vi "GetPulsePositionsByName.vi"(8 "error in (no error)":errorcluster, 10 "Channel Name":string, 11 "Pulse Positions Array":T1[](array[typedef])) -> (0 "error out":errorcluster, 1 "Pulse Positions":T1, 2 "Found?":bool, 3 "Pulse Positions Array Out":T1[](array[typedef]))   [LabVIEW 2017]
uses:
  <vilib>/addons/InsightCM/Utilities/Analysis/Shared/controls/PulsePositions.ctl
  <vilib>/addons/InsightCM/Utilities/Analysis/Shared/AnalysisHelper.lvlib
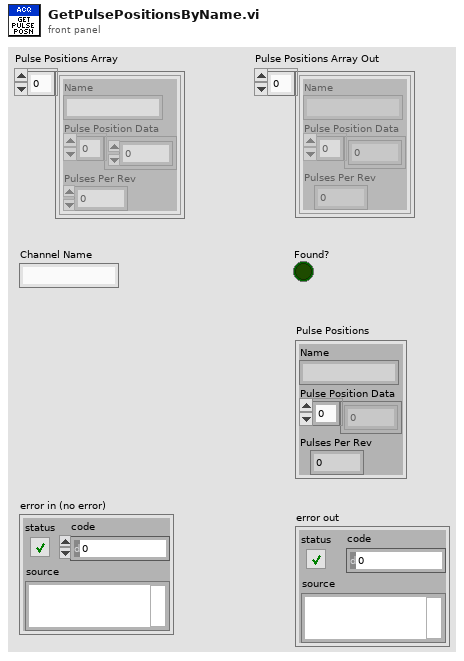
[diagram p1: front panel]
types:
  T1 = typedef "AnalysisHelper.lvlib/PulsePositions.ctl" = cluster{"Name":string, "Pulse Position Data":dbl[], "Pulses Per Rev":i32}
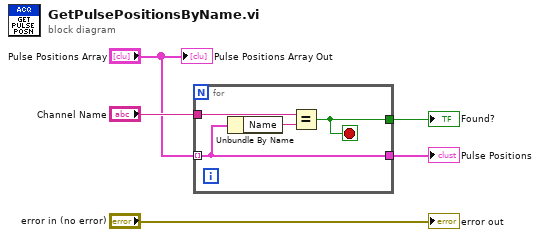
[diagram p0: block diagram]
diagram:
  n1 = for {
    tunnel: "Pulse Positions Array" -> [w7] mode=indexing
    tunnel: "Channel Name" -> [w9]
    tunnel: [w7] -> w1
    tunnel: [w8] -> w4
    stop <- w8 stop-if-true
    n2 = Unbundle By Name(w7) -> ("Name"=w6:string)
    n3 = Equal?(x=w9, y=w6) -> (x = y?=w8:bool)
  }
  "Found?" <- w4
  "Pulse Positions" <- w1
  "error out" <- "error in (no error)"
  "Pulse Positions Array Out" <- "Pulse Positions Array"
